vi "0-Read MDF.vi"(3 "MDF file":path) -> (1 "Waypoints List":T1)   [LabVIEW 2011]
doc: "Reads a MDF (Mission Definition File) as saved by 0-Save MDF.vi"
uses:
  0x2-OCU-Think Comm/0x2 Typedefs/Waypoints List.ctl
  0x2-OCU-Think Comm/0x2 Typedefs/ocuWaypoint.ctl
  0x2-OCU-Think Comm/0x2 Typedefs/waypointTypes.ctl
  2-Think/2 Typedefs/UTM Location.ctl
panel:
  out "substring before match":string
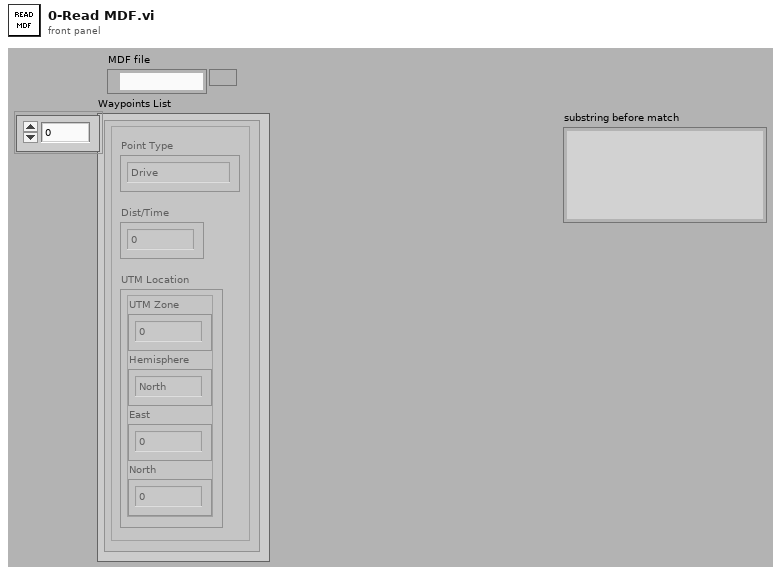
[diagram p1: front panel]
types:
  T1 = typedef "Waypoints List.ctl" = T2[]
  T2 = typedef "ocuWaypoint.ctl" = cluster{"Point Type":T3, "Dist/Time":dbl, "UTM Location":T4}
  T3 = typedef "waypointTypes.ctl" = enum16{"Drive", "Round Port", "Round Starboard", "Stay"}
  T4 = typedef "UTM Location.ctl" = cluster{"UTM Zone":dbl, "Hemisphere":enum16{"North", "South"}, "East":dbl, "North":dbl}
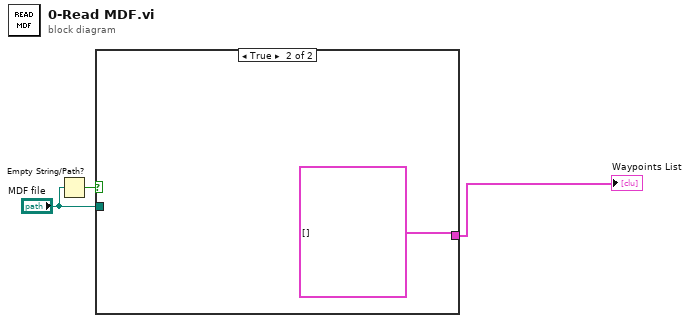
[diagram p0: block diagram]
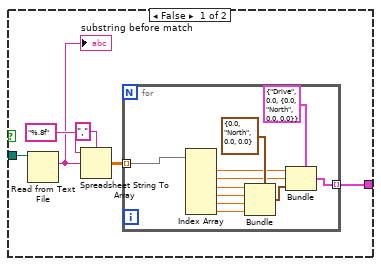
[diagram p2: hidden frame]
diagram:
  n1 = Empty String/Path?(string/path="MDF file") -> (empty?=w3:bool)
  n2 = case shown="True" w3 {
    tunnel: [w4 T1 [] ("Waypoints List 2")] -> w1
    tunnel: "MDF file" -> [w6 _]
    frame False {
      n3 = Read from Text File(file (use dialog)=w6) -> (text=w5:string)  [unwired: 3 in, 3 out]
      "substring before match" <- w5
      n4 = Spreadsheet String To Array(delimiter (Tab)=",", format string="%.8f", spreadsheet string=w5) -> (array=w7:dbl[][])  [unwired: 1 in]
      n5 = for {
        tunnel: w7 -> [w20] mode=indexing
        tunnel: [w19] -> w4 mode=indexing
        n6 = Index Array(array=w20) -> (element #1=w15:dbl, element #2=w14:dbl, element #3=w13:dbl, element #4=w12:dbl, element #5=w11:dbl, element #6=w10:dbl)  [unwired: 6 in]
        n7 = Bundle(cluster=T4 {"UTM Zone"=0.0, "Hemisphere"=enum."North", "East"=0.0, "North"=0.0} ("UTM Location"), "UTM Zone"=w13, "Hemisphere"=w12, "East"=w11, "North"=w10) -> (w16:T4)
        n8 = Bundle(cluster=T2 {"Point Type"=enum."Drive", "Dist/Time"=0.0, "UTM Location"={"UTM Zone"=0.0, "Hemisphere"=enum."North", "East"=0.0, "North"=0.0}} ("Waypoint"), "Point Type"=w15, "Dist/Time"=w14, "UTM Location"=w16) -> (w19:T2)
      }
    }
    frame True {
    }
  }
  "Waypoints List" <- w1
